vi "Get Deadband.vi"(8 "error in":errorcluster, 11 "TE Cooler in":refnum<class "TE Cooler.lvclass">) -> (0 "error out":errorcluster, 2 "Deadband":sgl, 3 "TE Cooler out":refnum<class "TE Cooler.lvclass">)   [LabVIEW 2014, in "TE Cooler.lvlib" / "TE Cooler.lvclass"]
doc: "Retrieve the controller deadband setting in the working units of the controller."
uses:
  TE Cooler.lvclass
  Controls/Command.ctl
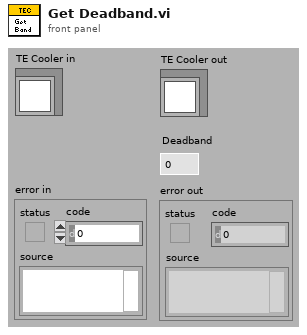
[diagram p1: front panel]
types:
  T1 = typedef "TE Cooler.lvlib/TE Cooler.lvclass/Command.ctl" = enum16{"INPUT1", "DESIRED CONTROL VALUE", "POWER OUTPUT", "ALARM STATUS", "INPUT 2", "OUTPUT CURRENT COUNTS", "ALARM TYPE", "SET TYPE DEFINE", "SENSOR TYPE", "CONTROL TYPE", "CONTROL OUTPUT POLARITY", "POWER ON/OFF", "OUTPUT SHUTDOWN IF ALARM", "FIXED DESIRED CONTROL SETTING", "PROPORTIONAL BANDWIDTH", "INTEGRAL GAIN", "DERIVATIVE GAIN", "LOW EXTERNAL SET RANGE", "HIGH EXTERNAL SET RANGE", "ALARM DEADBAND", "HIGH ALARM SETTING", "LOW ALARM SETTING", "CONTROL DEADBAND SETTING", "INPUT1 OFFSET", "INPUT2 OFFSET", "HEAT MULTIPLIER", "COOL MULTIPLIER", "OVER CURRENT COUNT COMPARE VALUE", "ALARM LATCH ENABLE", "NOT USED", "ALARM LATCH RESET", "CHOOSE SENSOR FOR ALARM FUNCTION", "CHOOSE TEMPERATURE WORKING UNITS", "EEPROM WRITE ENABLE", "OVER CURRENT CONTINUOUS", "OVER CURRENT RESTART ATTEMPTS", "JP3 DISPLAY ENABLE"}
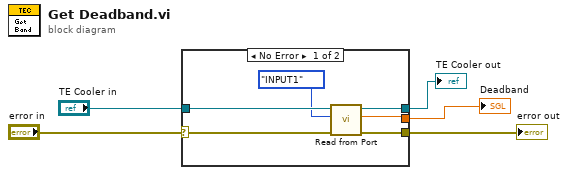
[diagram p0: block diagram]
diagram:
  n1 = case shown="No Error" "error in" {
    selector: "error in" -> [w9 w13]
    tunnel: [w8 w13] -> w4
    tunnel: [w10 w12] -> w2
    tunnel: "TE Cooler in" -> [w11 w12]
    tunnel: [w7 _] -> w1
    frame No Error {
      n2 = call "Read from Port.vi"("error in"=w9, "TEC Cmd"=Command."INPUT1", "TE Cooler in"=w11) -> ("error out"=w8:errorcluster, "scaledOut"=w7:sgl, "TE Cooler out"=w10:refnum<class "TE Cooler.lvclass">)  [unwired: 5 in, 1 out]
    }
    frame Error {
    }
  }
  "error out" <- w4
  "TE Cooler out" <- w2
  "Deadband" <- w1
